vi "Get Valid Channel Value String.vi"(9 "Previous Values":string, 11 "Channel Values":string) -> (3 "Valid Channel Values":string)   [LabVIEW 2020, in "Output Sequencer.lvlib" / "Settings UI.lvclass"]
uses:
  Settings UI.lvclass
  <vilib>/LAVA/muParser/mupExpr/mupExpr.lvclass
  <vilib>/Utility/error.llb/Trim Whitespace One-Sided.vi
  Output Sequencer/Globals/Global Strings.vi
  Globals/Dialog Strings.vi
  Output Sequencer/Output Sequencer.lvclass
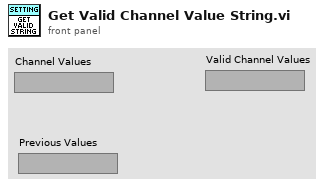
[diagram p1: front panel]
types:
  T1 = cluster{"error code":i32, "error message":string, "error pos":i32, "error token":string}
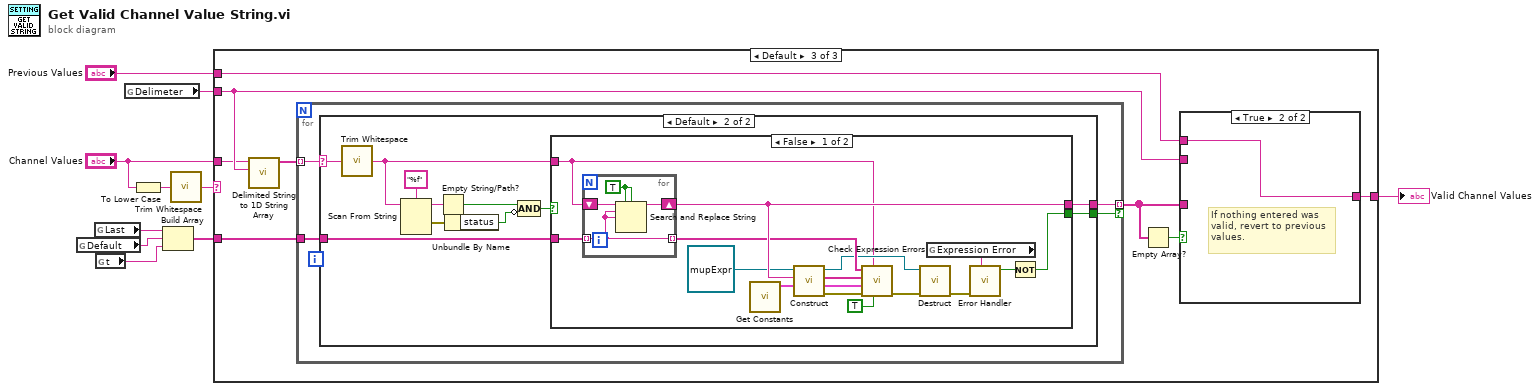
[diagram p0: block diagram]
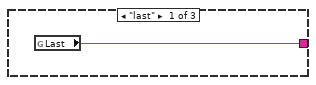
[diagram p2: hidden frame]
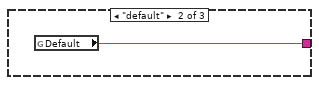
[diagram p3: hidden frame]
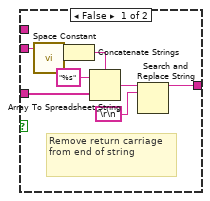
[diagram p4: hidden frame]
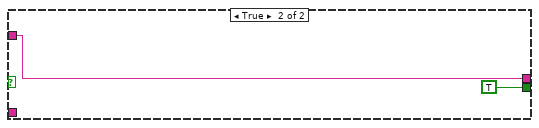
[diagram p6: hidden frame]
diagram:
  n1 = global read "Global Strings.vi" "Default"() -> (w4:string)
  n2 = global read "Global Strings.vi" "Last"() -> (w5:string)
  n3 = global read "Global Strings.vi" "t"() -> (w2:string)
  n4 = global read "Global Strings.vi" "Delimeter"() -> (w8:string)
  n5 = To Lower Case(string="Channel Values") -> (all lower case string=w7:string)
  n6 = Build Array(w5, w4, w2) -> (w3:string[])
  n7 = call <vilib>:"Trim Whitespace.vi"("string"=w7) -> ("trimmed string"=w6:string)  [unwired: 1 in]
  n8 = case shown="Default" w6 {
    tunnel: [w11 w12 w20] -> w9
    tunnel: w8 -> [_ _ w19]
    tunnel: "Channel Values" -> [_ _ w18]
    tunnel: w3 -> [_ _ w17]
    tunnel: "Previous Values" -> [_ _ w16]
    frame "last" {
      n9 = global read "Global Strings.vi" "Last"() -> (w11:string)
    }
    frame "default" {
      n10 = global read "Global Strings.vi" "Default"() -> (w12:string)
    }
    frame Default {
      n11 = call <vilib>:"Delimited String to 1D String Array.vi"("delimiter"=w19, "delimited string"=w18) -> ("string array"=w15:string[])  [unwired: 9 in]
      n12 = for {
        tunnel: w15 -> [w30] mode=indexing
        tunnel: [w33] -> w13 mode=indexing if=w32
        tunnel: w17 -> [w31]
        n13 = case shown="Default" w30 {
          selector: w30 -> [_ w34]
          tunnel: [_ w44] -> w33
          tunnel: [_ w43] -> w32
          tunnel: w31 -> [_ w42]
          frame "" {
          }
          frame Default {
            n14 = call <vilib>:"Trim Whitespace.vi"("string"=w34) -> ("trimmed string"=w35:string)  [unwired: 1 in]
            n15 = Scan From String(format string="%f", input string=w35) -> (remaining string=w40:string, error out=w39:errorcluster)  [unwired: 4 in, 1 out]
            n16 = Empty String/Path?(string/path=w40) -> (empty?=w38:bool)
            n17 = Unbundle By Name(w39) -> ("status"=w37:bool)
            n18 = Compound Arithmetic op=AND(w38, invert w37) -> (w36:bool)
            n19 = case shown="False" w36 {
              tunnel: [w58 w65] -> w44
              tunnel: [w59 TRUE] -> w43
              tunnel: w42 -> [w60 _]
              tunnel: w35 -> [w49 w65]
              frame False {
                n20 = for {
                  tunnel: w60 -> [w61] mode=indexing
                  tunnel: [w61] -> w51 mode=indexing
                  shift-right: [w62] -> w58
                  shift-left: w49 -> [w63]
                  w64 = TRUE ("replace all? (F)")
                  n21 = Search and Replace String(replace all?=w64, case sensitive?=w64, input string=w63, search string=w61, replace string=w61) -> (result string=w62:string)  [unwired: 3 in, 3 out]
                }
                n22 = call "Get Constants.vi"() -> ("Constants"=w56:cluster{"name":string, "value":dbl}[])  [unwired: 11 in]
                n23 = call-dynamic "Construct.vi"("Constants"=w56, "Expression"=w58, "muExpr in"=refnum<class "mupExpr.lvclass"> refnum) -> ("error out"=w55:errorcluster, "error details"=w52:T1, "Variable Names"=w53:string[], "mupExpr out"=w50:refnum<class "mupExpr.lvclass">)  [unwired: 5 in]
                n24 = call "Check Expression Errors.vi"("For dialog?"=TRUE, "Expression String in"=w49, "error in (no error)"=w55, "Parser Error Details"=w52, "Found Variables"=w53, "Expected Variables"=w51) -> ("error out"=w54:errorcluster)  [unwired: 5 in]
                n25 = call-dynamic "Destruct.vi"("error in (no error)"=w54, "muExpr in"=w50) -> ("error out"=w47:errorcluster)  [unwired: 9 in]
                n26 = global read "Dialog Strings.vi" "Expression Error"() -> (w48:string)
                n27 = call "Error Handler.vi"("Dialog Title (\"\")"=w48, "error in (no error)"=w47) -> ("Error?"=w46:bool)  [unwired: 9 in]
                n28 = Not(x=w46) -> (.not. x?=w59:bool)
              }
              frame True {
              }
            }
          }
        }
      }
      n29 = Empty Array?(array=w13) -> (empty?=w14:bool)
      n30 = case shown="True" w14 {
        tunnel: w13 -> [w28 _]
        tunnel: w19 -> [w24 _]
        tunnel: [w25 w29] -> w20
        tunnel: w16 -> [_ w29]
        frame False {
          # "Remove return carriage from end of string"
          n31 = call <vilib>:"Space Constant.vi"() -> ("String"=w23:string)
          n32 = Concatenate Strings(w24, w23) -> (w22:string)
          n33 = Array To Spreadsheet String(delimiter (Tab)=w22, array=w28, 3:"%s" ("format string")) -> (spreadsheet string=w27:string)
          n34 = Search and Replace String(input string=w27, search string="\r\n") -> (result string=w25:string)  [unwired: 6 in, 3 out]
        }
        frame True {
          # "If nothing entered was\nvalid, revert to previous\nvalues."
        }
      }
    }
  }
  "Valid Channel Values" <- w9
